vi "Test Draw.vi"(11 "Test Case In":refnum<class "Sprite Font Tests.lvclass">) -> (0 "error out":errorcluster, 3 "Test Case Out":refnum<class "Sprite Font Tests.lvclass">)   [LabVIEW 2021, in "Sprite Font Tests.lvclass"]
uses:
  Sprite Font Tests.lvclass
  C:/Program Files (x86)/National Instruments/LabVIEW 2026/vi.lib/Astemes/LUnit/Test Case.lvclass
  <vilib>/Astemes/LUnit/Test Case.lvclass/Test Case.ctl
  Application Specific/Renderer/Renderer.lvclass
  Application Specific/Sprite Font/Sprite Font.lvclass
  Application Specific/Resource Manager/Resource Manager.lvclass
  LabSDL2/Source/Libraries/LibSDL2 Wrapper/LibSDL2.lvlib
  LabSDL2/Source/Libraries/LibSDL2 Wrapper/Controls/Rectangle.ctl
  Application Specific/Sprite Font/Game Font.ctl
  <vilib>/Astemes/LUnit/Test Case.lvclass
  Re-use Libraries/Vector 2D/Vector 2D.lvclass
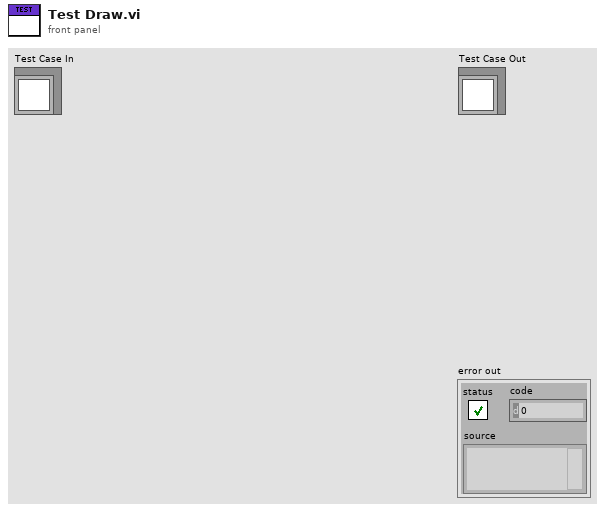
[diagram p1: front panel]
types:
  T1 = typedef "Sprite Font.lvclass/Game Font.ctl" = enum16{"Ilwrath", "Micro", "Slylandro", "Starcon", "Tiny", "Utwig"}
  T2 = typedef "LibSDL2.lvlib/Rectangle.ctl" = cluster{"x":i32, "y":i32, "Width":i32, "Height":i32}
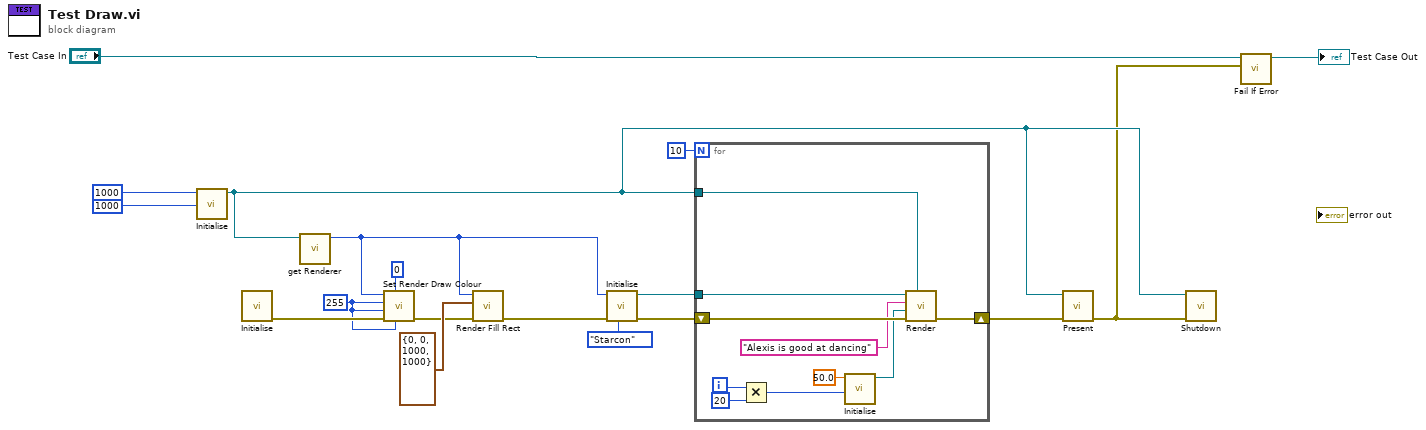
[diagram p0: block diagram]
diagram:
  w7 = u8 255 ("R")
  n1 = call "Initialise.vi"("Window Height"=1000 ("Height"), "Window Width"=1000 ("Width")) -> ("Renderer out"=w13:refnum<class "Renderer.lvclass">)  [unwired: 8 in, 1 out]
  n2 = call "Initialise.vi"() -> ("error out"=w10:errorcluster)  [unwired: 11 in]
  n3 = call-dynamic "get Renderer.vi"("Renderer in"=w13) -> ("Renderer"=w8:u32)  [unwired: 10 in]
  n4 = call "Set Render Draw Colour.vi"("B"=w7, "A"=u8 0, "error in (no error)"=w10, "G"=w7, "R"=w7, "Renderer Pointer"=w8) -> ("error out"=w9:errorcluster)  [unwired: 4 in, 1 out]
  n5 = call "Render Fill Rect.vi"("error in"=w9, "Rectangle"=T2 {"x"=0, "y"=0, "Width"=1000, "Height"=1000}, "Renderer Pointer"=w8) -> ("error out"=w12:errorcluster)  [unwired: 7 in, 1 out]
  n6 = call "Initialise.vi"("Font"=Game_Font."Starcon", "error in (no error)"=w12, "Renderer"=w8) -> ("error out"=w15:errorcluster, "Font out"=w16:refnum<class "Sprite Font.lvclass">)  [unwired: 7 in]
  n7 = for {
    N: 10 -> [_]
    tunnel: w16 -> [w28]
    tunnel: w13 -> [w25]
    shift-right: [w26] -> w14
    shift-left: w15 -> [w27]
    i -> [w21]
    n8 = Multiply(x=w21, y=20) -> (x*y=w19:i32)
    n9 = call "Initialise.vi"("y"=w19, "x"=sgl 50.0) -> ("Vector 2D out"=w23:refnum<class "Vector 2D.lvclass">)  [unwired: 9 in]
    n10 = call-dynamic "Render.vi"("Renderer"=w25, "error in (no error)"=w27, "Position"=w23, "String"="Alexis is good at dancing", "Font in"=w28) -> ("error out"=w26:errorcluster)  [unwired: 6 in]
  }
  n11 = call "Present.vi"("error in (no error)"=w14, "Renderer"=w13) -> ("error out"=w3:errorcluster)  [unwired: 9 in]
  n12 = call "Shutdown.vi"("error in (no error)"=w3, "Renderer"=w13) -> ()  [unwired: 9 in, 1 out]
  n13 = call <vilib>:"Fail If Error.vi"("Assert error"=w3, "LUnit Test Case In"="Test Case In") -> ("LUnit Test Case Out"=→"Test Case Out":refnum<class "Sprite Font Tests.lvclass">)  [unwired: 8 in, 1 out]
